vi "Extract Item Names.vi"(3 "Step Array":T1[](array[typedef])) -> (1 "Item Names":string[][](array[string]))   [LabVIEW 2018]
uses:
  type defs/Sequence Info.ctl
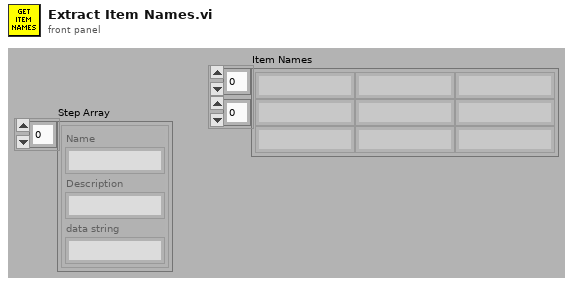
[diagram p1: front panel]
types:
  T1 = typedef "Sequence Info.ctl" = cluster{"Name":string, "Description":string, "data string":string}
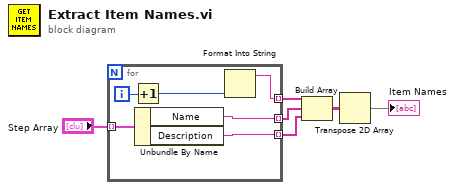
[diagram p0: block diagram]
diagram:
  n1 = for {
    tunnel: "Step Array" -> [w12] mode=indexing
    tunnel: [w9] -> w3 mode=indexing
    tunnel: [w8] -> w2 mode=indexing
    tunnel: [w7] -> w1 mode=indexing
    i -> [w10]
    n2 = Increment(x=w10) -> (x+1=w11:i32)
    n3 = Unbundle By Name(w12) -> ("Name"=w8:string, "Description"=w7:string)
    n4 = Format Into String(w11) -> (resulting string=w9:string)  [unwired: 3 in, 1 out]
  }
  n5 = Build Array(w3, w2, w1) -> (w5:string[][])
  n6 = Transpose 2D Array(2D array=w5) -> (transposed array=→"Item Names":string[][])
